vi "AFT Create FIR Fast Block LMS.vi"(8 "error in (no error)":errorcluster, 9 "constrained? (T)":bool=TRUE, 10 "step size":dbl=0.01, 11 "filter length":i32=128) -> (0 "error out":errorcluster, 3 "adaptive filter out":refnum<k20>)   [LabVIEW 2017, in "NI_AdaptiveFilter.lvlib"]
doc: "Creates a finite impulse response (FIR) adaptive filter with the fast block least mean squares (LMS) algorithm."
uses:
  <vilib>/addons/Adaptive Filters/NI_AdaptiveFilter.lvlib
  <resource>/AdaptiveFilters.dll
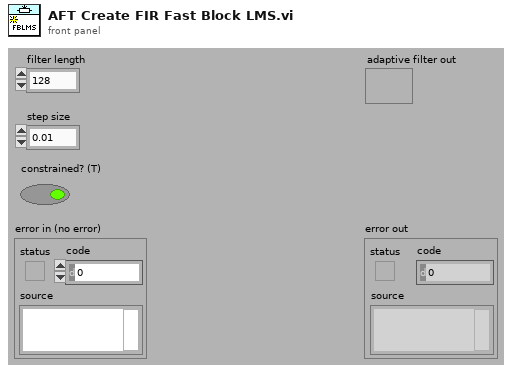
[diagram p1: front panel]
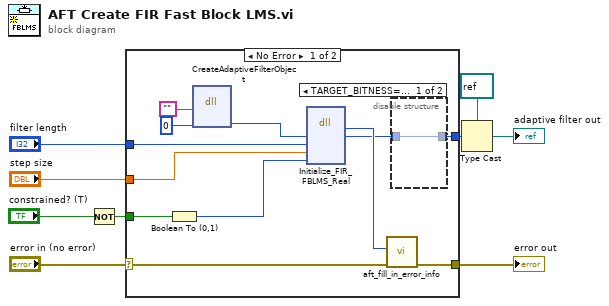
[diagram p0: block diagram]
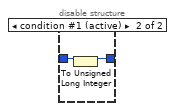
[diagram p2: hidden frame]
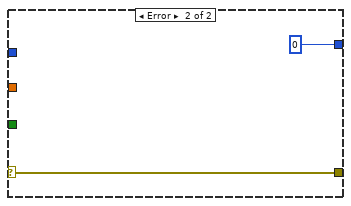
[diagram p3: hidden frame]
diagram:
  n1 = Not(x="constrained? (T)") -> (.not. x?=w1:bool)
  n2 = case shown="No Error" "error in (no error)" {
    selector: "error in (no error)" -> [w15 w26]
    tunnel: [w14 w26] -> w8
    tunnel: "filter length" -> [w18 _]
    tunnel: "step size" -> [w17 _]
    tunnel: [w10 u32 0 ("pSession")] -> w5
    tunnel: w1 -> [w13 _]
    frame No Error {
      n3 = Boolean To (0,1)(Boolean=w13) -> (0, 1=w12:i16)
      n4 = dll-call lib="C:/Program Files/National Instruments/LabVIEW 2017/resource/AdaptiveFilters.*" fn="CreateAdaptiveFilterObject" ("Complex Data Create")("UnusedReferenceName"="", "pConfigurationHandle"=u32 0 ("pScriptRefNum")) -> ("pConfigurationHandle"=w19:u64)  [unwired: 3 in, 4 out]
      n5 = dll-call lib="C:/Program Files/National Instruments/LabVIEW 2017/resource/AdaptiveFilters.*" fn="Initialize_FIR_FBLMS_Real" ("Complex Data Initialization")("pSession"=w19, "order"=w18, "mu"=w17, "unconstrained"=w12) -> ("err"=w16:i32, "pSession"=w11:u64)  [unwired: 6 in, 2 out]
      n6 = call <vilib>:"aft_fill_in_error_info.vi"("error in"=w15, "status code"=w16) -> ("error out"=w14:errorcluster)  [unwired: 2 in, 7 out]
      n7 = disable-structure shown="TARGET_BITNESS==64, Default" {
        disable-tunnel: w11 -> [w22 w24]
        disable-tunnel: [w22 w23] -> w10
        frame condition #0 {
        }
        frame condition #1 (active) {
          n8 = To Unsigned Long Integer(number=w24) -> (unsigned 32bit integer=w23:u32)
        }
      }
    }
    frame Error {
    }
  }
  "error out" <- w8
  n9 = Type Cast(type=refnum<k20> refnum ("filtered-x in 4"), x=w5) -> (*(type *) &x=→"adaptive filter out":refnum<k20>)
